vi "stop_scanning.vi"(8 "error in (no error)":errorcluster, 11 "ScanModeDL090923Scaffold in":refnum<class "ImagingModeDL090923Scaffold.lvclass">) -> (0 "error out":errorcluster, 3 "ScanModeDL090923Scaffold out":refnum<class "ImagingModeDL090923Scaffold.lvclass">)   [LabVIEW 2010, in "ImagingModeDL090923Scaffold.lvclass"]
uses:
  ImagingModeDL090923Scaffold.lvclass
  common/classes/ErrorController/ErrorController/class_data.vi
  ScanHead/GenericScanHead/GenericScanHead/GenericScanHead.lvclass
  DAQ/GenericDAQ/GenericDAQ/GenericDAQ.lvclass
  common/classes/ErrorController/ErrorController/ErrorController.lvclass
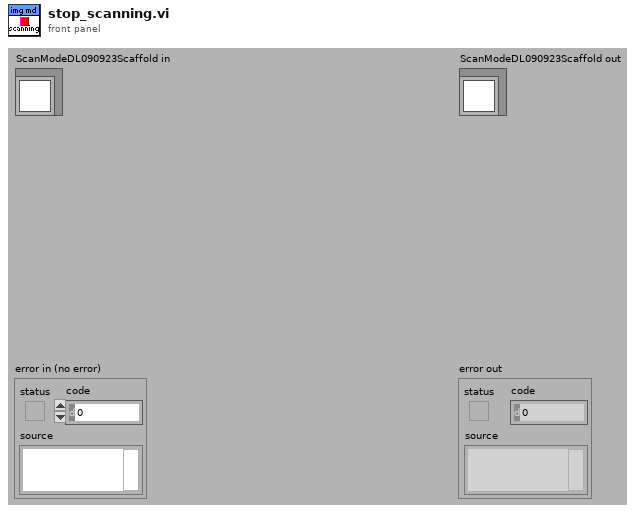
[diagram p1: front panel]
types:
  T1 = typedef "GenericToplevelComponent.lvclass/common_trigger_enum.ctl" = enum16{"NULL", "initialise", "terminate", "fetch command", "fetch data", "attach observer", "register as observer", "detach observer", "acknowledge", "start", "stop", "sweep started", "sweep finished", "experiment started", "experiment stopped"}
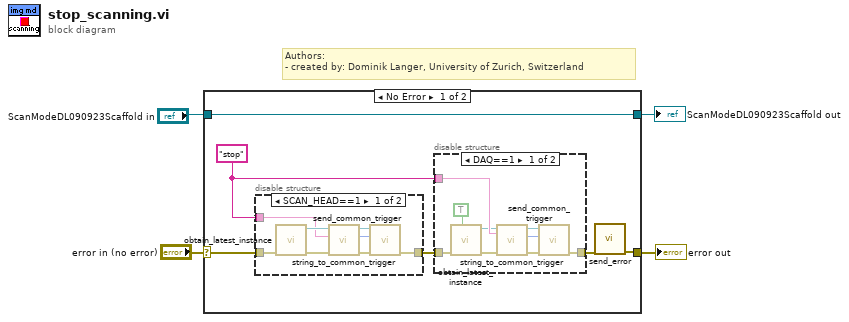
[diagram p0: block diagram]
diagram:
  # "Authors: \n- created by: Dominik Langer, University of Zurich, Switzerland"
  n1 = case shown="No Error" "error in (no error)" {
    selector: "error in (no error)" -> [w9 w31]
    tunnel: [w7 w31] -> w1
    tunnel: [w10 w30] -> w4
    tunnel: "ScanModeDL090923Scaffold in" -> [w10 w30]
    frame No Error {
      w5 = "stop"
      n2 = disable-structure shown="SCAN_HEAD==1" {
        disable-tunnel: w9 -> [w27 w29]
        disable-tunnel: [w28 w29] -> w8
        disable-tunnel: w5 -> [w21 _]
        frame condition #0 {
          n3 = call "obtain_latest_instance.vi"("error in (no error)"=w27) -> ("error out"=w25:errorcluster, "GenericScanHead out"=w26:refnum<class "GenericScanHead.lvclass">)  [unwired: 1 in, 8 out]
          n4 = call-dynamic "string_to_common_trigger.vi"("error in (no error)"=w25, "trigger string"=w21, "GenericToplevelComponent in"=w26) -> ("error out"=w24:errorcluster, "trigger"=w22:T1, "GenericToplevelComponent out"=w23:refnum<class "GenericScanHead.lvclass">)  [unwired: 6 in]
          n5 = call-dynamic "send_common_trigger.vi"("error in (no error)"=w24, "trigger"=w22, "GenericToplevelComponent in"=w23) -> ("error out"=w28:errorcluster)  [unwired: 6 in, 2 out]
        }
        frame condition #1 (active) {
        }
      }
      n6 = disable-structure shown="DAQ==1" {
        disable-tunnel: w8 -> [w18 w20]
        disable-tunnel: [w19 w20] -> w6
        disable-tunnel: w5 -> [w14 _]
        frame condition #0 {
          n7 = call "obtain_latest_instance.vi"("quick, but maybe outdated?"=TRUE, "error in (no error)"=w18) -> ("error out"=w16:errorcluster, "GenericDAQ out"=w13:refnum<class "GenericDAQ.lvclass">)  [unwired: 8 out]
          n8 = call-dynamic "string_to_common_trigger.vi"("error in (no error)"=w16, "trigger string"=w14, "GenericToplevelComponent in"=w13) -> ("error out"=w15:errorcluster, "trigger"=w11:T1, "GenericToplevelComponent out"=w12:refnum<class "GenericDAQ.lvclass">)  [unwired: 6 in]
          n9 = call-dynamic "send_common_trigger.vi"("error in (no error)"=w15, "trigger"=w11, "GenericToplevelComponent in"=w12) -> ("error out"=w19:errorcluster)  [unwired: 6 in, 2 out]
        }
        frame condition #1 (active) {
        }
      }
      n10 = call "send_error.vi"("error in (no error)"=w6) -> ("error out"=w7:errorcluster)  [unwired: 10 in]
    }
    frame Error {
    }
  }
  "error out" <- w1
  "ScanModeDL090923Scaffold out" <- w4
